vi "Main.vi"(11 "Module Admin":refnum<class "Delacor_lib_QMH_Cloneable Module Admin.lvclass">) -> ()   [LabVIEW 2020, in "Client HTTP Post.lvlib"]
doc: "This template is based off of the Queued Message Handler design pattern and the Queued Message Handler project template that ships with LabVIEW.\n\nThe main difference is that the queue is private to this module and communication between modules is performed via Broadcast and Request events.\n\nRequest events are wrapped in public API methods and are handled in the Event Handling Loop (EHL) of this VI. Any module can register for Broadcast events sent by this module. The EHL generates messages based on user interface actions.\n\nThe Message Handling Loop (MHL) processes messages generated by the EHL, or by other messages. The messages are string values, so new messages can be added easily to the Message Cases case structure in the MHL. Each message cluster can also provide an optional value for Message Data, which is a variant that can be converted to whatever message-specific data is required.\n_____\nBased on DQMH Project Template 6.0.0.91."
uses:
  Client HTTP Post.lvlib
  <vilib>/Delacor/Delacor QMH/Libraries/Cloneable Module Admin_class/Delacor_lib_QMH_Cloneable Module Admin.lvclass
  C:/Program Files (x86)/National Instruments/LabVIEW 2020/vi.lib/Delacor/Delacor QMH/Libraries/Module Admin_class/Delacor_lib_QMH_Module Admin.lvclass
  Module Data--cluster.ctl
  Do Something Argument--cluster.ctl
  <vilib>/Delacor/Delacor QMH/Libraries/Message Queue_class/Delacor_lib_QMH_Message Queue.lvclass/Delacor_lib_QMH_Message Queue.ctl
  Do Something Else Argument--cluster.ctl
  Do Something Else and Wait for Reply Argument--cluster.ctl
  Do Something Else and Wait (Reply Payload)--cluster.ctl
  <vilib>/Delacor/Delacor QMH/Libraries/Cloneable Module Admin_class/Delacor_lib_QMH_Cloneable Module Admin.lvclass/Delacor_lib_QMH_Cloneable Module Admin.ctl
  Stop Argument--cluster.ctl
  <vilib>/Delacor/Delacor QMH/Libraries/Module Admin_class/Delacor_lib_QMH_Module Admin.lvclass/Delacor_lib_QMH_Module Admin.ctl
  <vilib>/Delacor/Delacor QMH/Libraries/Message Queue_class/Delacor_lib_QMH_Enqueue Message (Single).vi
  <vilib>/Delacor/Delacor QMH/Libraries/Cloneable Module Admin_class/Delacor_lib_QMH_Get Module ID.vi
  <vilib>/Delacor/Delacor QMH/Libraries/Module Admin_class/Delacor_lib_QMH_Get External Launch.vi
  <vilib>/httpClient/POSTBuffer.vi
  <vilib>/Utility/error.llb/Error Cluster From Error Code.vi
  <vilib>/ErrorRing/Error Ring.xnode
  <vilib>/Delacor/Delacor QMH/Libraries/Message Queue_class/Delacor_lib_QMH_Message Queue.lvclass
  Hardware DAQ/Hardware DAQ.lvlib
  <vilib>/httpClient/LabVIEWHTTPClient.lvlib
panel:
  out "Array Data Termocuple & Voltage":dbl[](array[numeric])
  in  "Enviar":bool
  in  "Variables":enum16{"1 Variable", "Mas de una Variable"}(ring)
  out "body":string
  out "headers":string
  in  "POST":T1={"URL"="things.ubidots.com/api/v1.6/devices/system_daq", "Nombre - Variable"="signal", "Token"="BBFF-FQubfN2B9slUP8xWYB99mULTCcM9aX"}
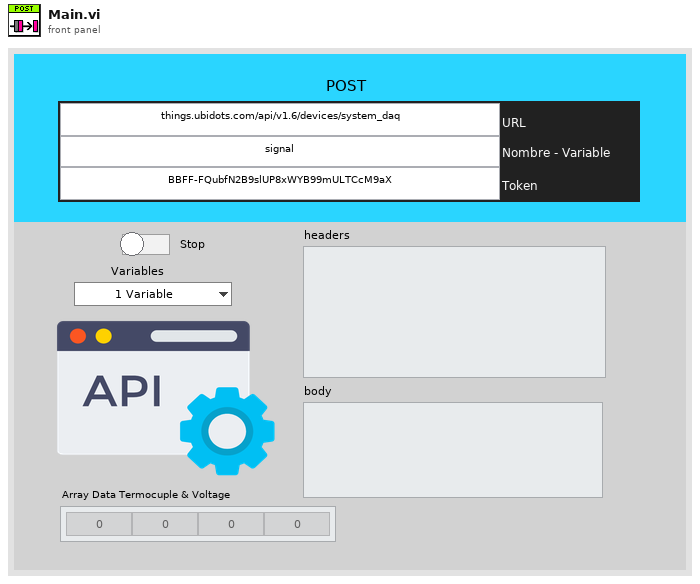
[diagram p1: front panel]
types:
  T1 = cluster{"URL":string, "Nombre - Variable":string, "Token":string}
  T2 = typedef "Client HTTP Post.lvlib/Request Events--cluster.ctl" = cluster{"Stop Module":refnum<user-event>, "Do Something":refnum<user-event>, "Do Something Else":refnum<user-event>, "Do Something Else and Wait for Reply":refnum<user-event>, "Show Panel":refnum<user-event>, "Hide Panel":refnum<user-event>, "Show Diagram":refnum<user-event>, "Get Module Execution Status":refnum<user-event>}
  T3 = typedef "Hardware DAQ.lvlib/Broadcast Events--cluster.ctl" = cluster{"Module Did Init":refnum<user-event>, "Status Updated":refnum<user-event>, "Error Reported":refnum<user-event>, "Module Did Stop":refnum<user-event>, "Update Module Execution Status":refnum<user-event>, "Hardware Connected":refnum<user-event>, "Data Process Volt":refnum<user-event>, "Coil values":refnum<user-event>}
  T4 = typedef "Client HTTP Post.lvlib/Module Data--cluster.ctl" = cluster{"Status":string}
  T5 = typedef "Client HTTP Post.lvlib/Do Something Argument--cluster.ctl" = cluster{"Module ID":i32, "Do Something Msg":string}
  T6 = typedef "Client HTTP Post.lvlib/Do Something Else Argument--cluster.ctl" = cluster{"Module ID":i32, "Do Something Else Msg":string, "X":dbl}
  T7 = typedef "Client HTTP Post.lvlib/Do Something Else and Wait for Reply Argument--cluster.ctl" = cluster{"Module ID":i32, "Do Something Else Msg":string, "X":dbl, "Wait Notifier":refnum<notifier>, "wait for reply":bool}
  T8 = enum32{"invalid lock state", "Not Locked", "Locked (No Password)", "Password-protected"}
  T9 = typedef "Client HTTP Post.lvlib/Stop Argument--cluster.ctl" = cluster{"Module ID":i32, "Origin":string, "Exit via Stop Module Req?":bool, "Wait for Module to stop?":bool}
  T10 = enum32{"Invalid", "Standard", "Closed", "Hidden", "Minimized", "Maximized"}
  T11 = cluster{"POST":cluster{"URL":string, "Nombre - Variable":string, "Token":string}, "Data Process.Volt":dbl[]}
  T12 = typedef "Client HTTP Post.lvlib/Do Something Else and Wait (Reply Payload)--cluster.ctl" = cluster{"Value":dbl, "error":errorcluster}
  T13 = typedef "LabVIEWHTTPClient.lvlib/ClientHandle.ctl" = refnum<k1>
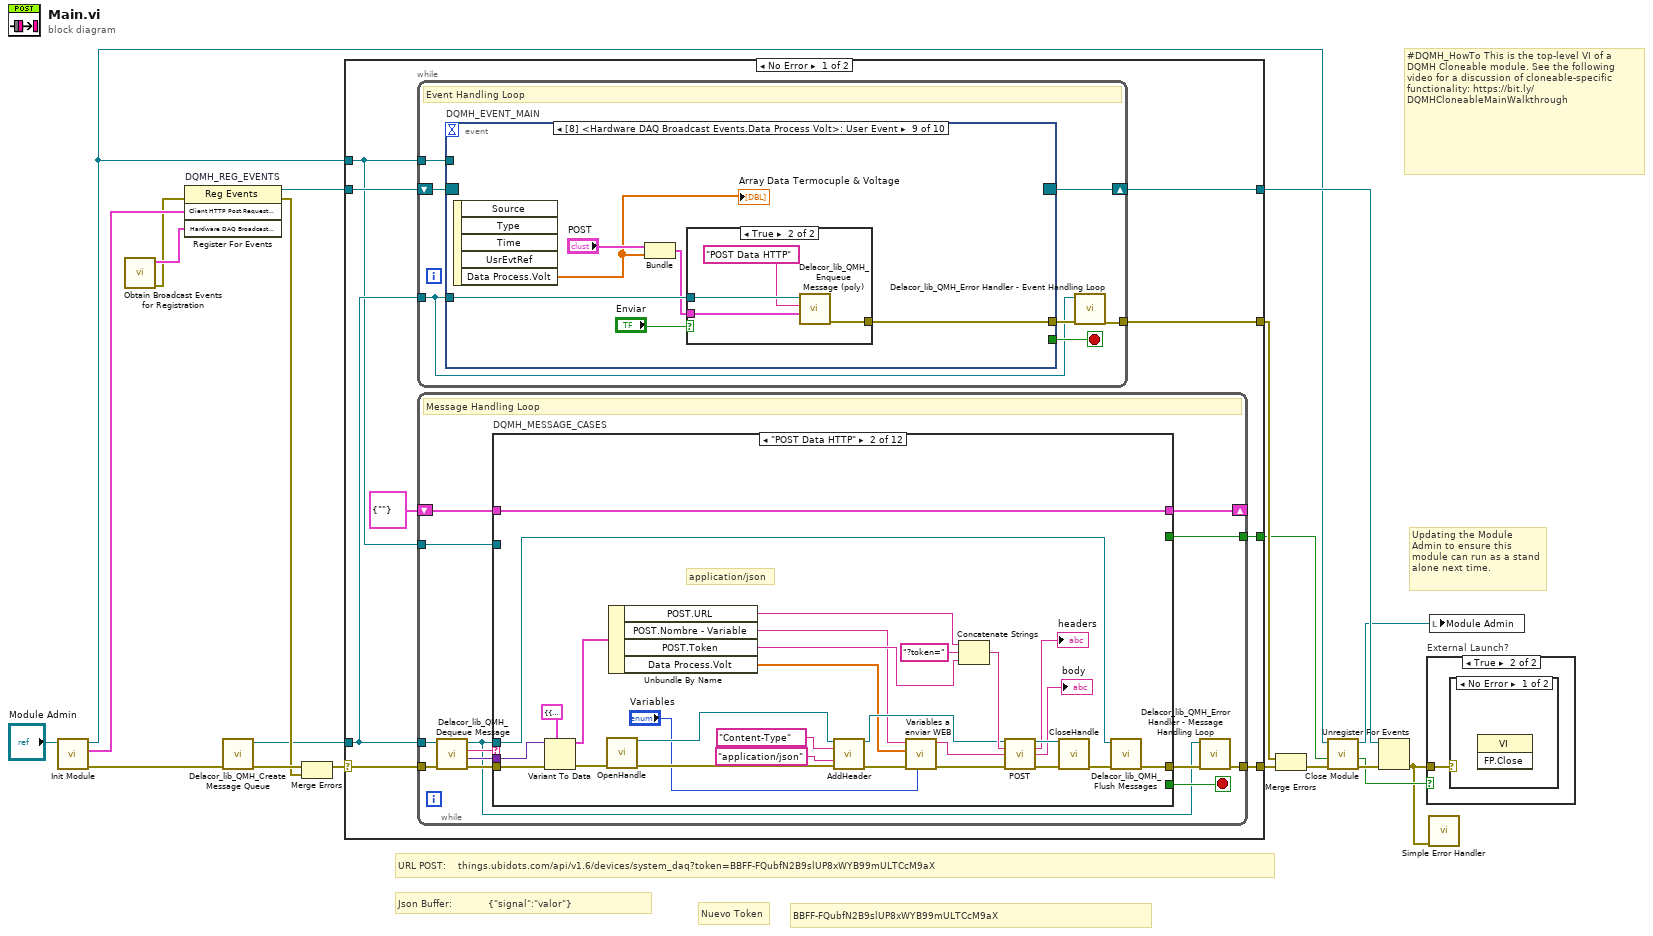
[diagram p0: block diagram]
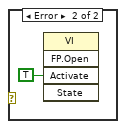
[diagram p3: hidden frame]
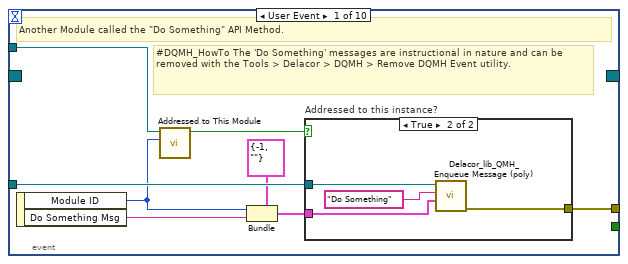
[diagram p4: hidden frame]
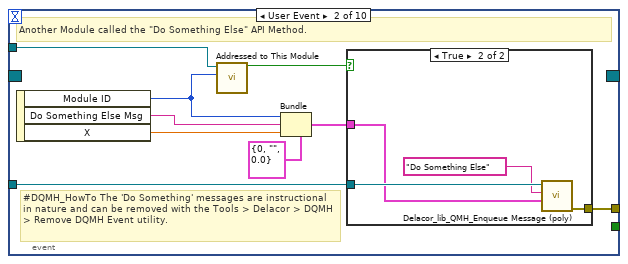
[diagram p6: hidden frame]
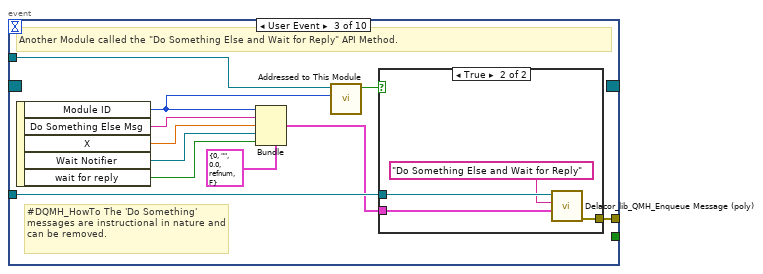
[diagram p8: hidden frame]
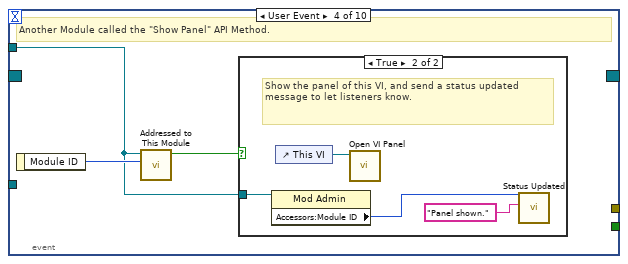
[diagram p10: hidden frame]
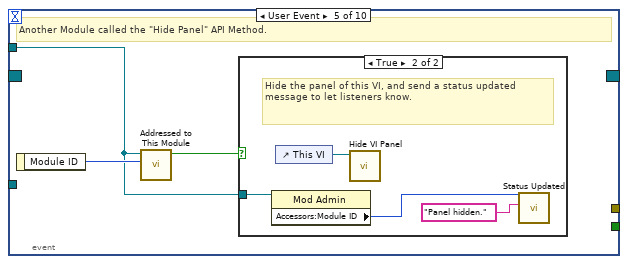
[diagram p12: hidden frame]
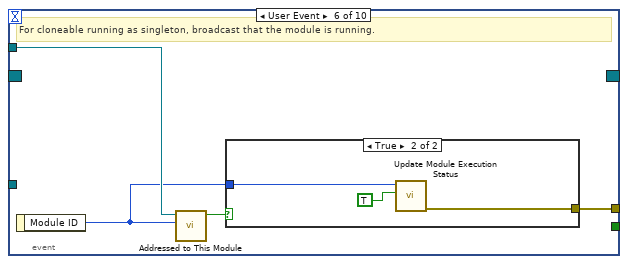
[diagram p14: hidden frame]
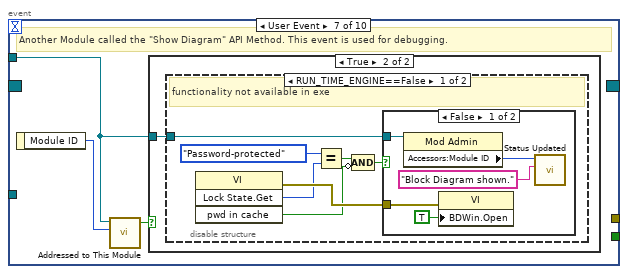
[diagram p16: hidden frame]
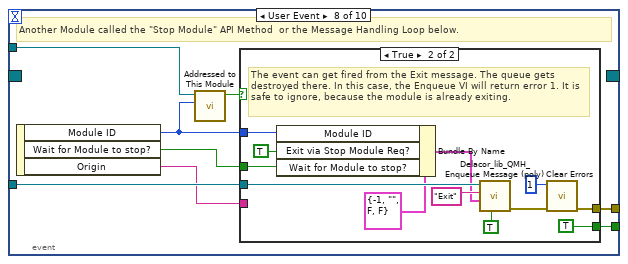
[diagram p20: hidden frame]
diagram:
  # "BBFF-FQubfN2B9slUP8xWYB99mULTCcM9aX"
  # "Nuevo Token"
  # "URL POST:    things.ubidots.com/api/v1.6/devices/system_daq?token=BBFF-FQubfN2B9slUP8xWYB99mULTCcM9aX"
  # "Json Buffer:            {\"signal\":\"valor\"}"
  # "#DQMH_HowTo This is the top-level VI of a DQMH Cloneable module. See the following video for a discussion of cloneable-specific functionality: https://bit.ly/DQMHCloneableMainWalkthrough"
  # "Updating the Module Admin to ensure this module can run as a stand alone next time."
  n1 = call "Init Module.vi"("Cloneable Module Admin in"="Module Admin") -> ("error out"=w17:errorcluster, "Client HTTP Post Request Events"=w10:T2, "Cloneable Module Admin out"=w7:refnum<class "Delacor_lib_QMH_Cloneable Module Admin.lvclass">)  [unwired: 8 in]
  n2 = call "Obtain Broadcast Events for Registration.vi"() -> ("error out"=w1:errorcluster, "Hardware DAQ Broadcast Events"=w2:T3)  [unwired: 9 in, 1 out]
  n3 = register-events "DQMH_REG_EVENTS"(error in=w1, w10, w2) -> (reference out=w11:refnum<event-registration>, error out=w13:errorcluster)  [unwired: 1 in]
  n4 = call <vilib>:"Delacor_lib_QMH_Create Message Queue.vi"("error in"=w17) -> ("error out"=w15:errorcluster, "Message Queue"=w9:refnum<class "Delacor_lib_QMH_Message Queue.lvclass">)  [unwired: 9 in]
  n5 = Merge Errors(w15, w13) -> (w14:errorcluster)
  n6 = case shown="No Error" w14 {
    selector: w14 -> [w27 w338]
    tunnel: [w29 w337] -> w18
    tunnel: [w26 w345] -> w12
    tunnel: w11 -> [w24 w345]
    tunnel: w9 -> [w23 w336]
    tunnel: [w28 _] -> w19
    tunnel: w7 -> [w22 w341]
    tunnel: [w21 _] -> w5
    frame No Error {
      n7 = while {
        tunnel: w23 -> [w30]
        shift-right: [w33] -> w26
        shift-left: w24 -> [w34]
        tunnel: [w35] -> w28
        tunnel: w22 -> [w31]
        stop <- w32 stop-if-true
        # "Event Handling Loop"
        n8 = event "DQMH_EVENT_MAIN" shown="[8] <Hardware DAQ Broadcast Events.Data Process Volt>: User Event" {
          selector: w34 -> [_ _ _ _ _ _ _ _ _ _]
          dyn-events: [_ _ _ _ _ _ _ _ _ _] -> w33
          timeout: _ -> [_ _ _ _ _ _ _ _ _ _]
          tunnel: [_ _ _ _ _ _ _ w117 _ _] -> w32
          tunnel: w30 -> [w43 w56 w71 _ _ _ _ w120 w139 w146]
          tunnel: [w44 w57 w72 _ _ w94 _ w121 w134 w149] -> w36
          tunnel: w31 -> [w41 w54 w69 w77 w84 w92 w98 w119 _ w147]
          event User Event {
            # "#DQMH_HowTo The 'Do Something' messages are instructional in nature and can be removed with the Tools > Delacor > DQMH > Remove DQMH Event utility."
            # "Another Module called the \"Do Something\" API Method."
            n9 = event-data() -> ("Module ID"=w38:i32, "Do Something Msg"=w37:string)  [unwired: 1 in]
            n10 = call "Addressed to This Module.vi"("Module ID from Argument"=w38, "Module Admin"=w41) -> ("Addressed to this instance?"=w42:bool)  [unwired: 8 in, 1 out]
            n11 = Bundle(cluster=T5 {"Module ID"=-1, "Do Something Msg"=""} ("Do Something Argument"), "Module ID"=w38, "Do Something Msg"=w37) -> (w40:T5)
            n12 = case "Addressed to this instance?" shown="True" w42 {
              tunnel: w43 -> [_ w47]
              tunnel: [_ w48] -> w44
              tunnel: w40 -> [_ w45]
              frame False {
                # "Do nothing"
              }
              frame True {
                n13 = call-poly <vilib>:"Delacor_lib_QMH_Enqueue Message (poly).vi"("Message Data"=w45, "Message"="Do Something", "Message Queue in"=w47) -> ("error out"=w48:errorcluster)  [unwired: 7 in, 1 out]
              }
            }
          }
          event User Event {
            # "#DQMH_HowTo The 'Do Something' messages are instructional in nature and can be removed with the Tools > Delacor > DQMH > Remove DQMH Event utility."
            # "Another Module called the \"Do Something Else\" API Method."
            n14 = event-data() -> ("Module ID"=w49:i32, "Do Something Else Msg"=w50:string, "X"=w52:dbl)  [unwired: 1 in]
            n15 = call "Addressed to This Module.vi"("Module ID from Argument"=w49, "Module Admin"=w54) -> ("Addressed to this instance?"=w55:bool)  [unwired: 8 in, 1 out]
            n16 = Bundle(cluster=T6 {"Module ID"=0, "Do Something Else Msg"="", "X"=0.0} ("Do Something Else Argument"), "Module ID"=w49, "Do Something Else Msg"=w50, "X"=w52) -> (w51:T6)
            n17 = case shown="True" w55 {
              tunnel: w56 -> [_ w60]
              tunnel: [_ w61] -> w57
              tunnel: w51 -> [_ w58]
              frame False {
              }
              frame True {
                n18 = call-poly <vilib>:"Delacor_lib_QMH_Enqueue Message (poly).vi"("Message Data"=w58, "Message"="Do Something Else", "Message Queue in"=w60) -> ("error out"=w61:errorcluster)  [unwired: 7 in, 1 out]
              }
            }
          }
          event User Event {
            # "#DQMH_HowTo The 'Do Something' messages are instructional in nature and can be removed."
            # "Another Module called the \"Do Something Else and Wait for Reply\" API Method."
            n19 = event-data() -> ("Module ID"=w67:i32, "Do Something Else Msg"=w65:string, "X"=w64:dbl, "Wait Notifier"=w63:refnum<notifier>, "wait for reply"=w62:bool)  [unwired: 1 in]
            n20 = Bundle(cluster=T7 {"Module ID"=0, "Do Something Else Msg"="", "X"=0.0, "Wait Notifier"=refnum, "wait for reply"=FALSE} ("Do Something Else and Wait for Reply Argument"), "Module ID"=w67, "Do Something Else Msg"=w65, "X"=w64, "Wait Notifier"=w63, "wait for reply"=w62) -> (w66:T7)
            n21 = call "Addressed to This Module.vi"("Module ID from Argument"=w67, "Module Admin"=w69) -> ("Addressed to this instance?"=w70:bool)  [unwired: 8 in, 1 out]
            n22 = case shown="True" w70 {
              tunnel: [_ w76] -> w72
              tunnel: w71 -> [_ w75]
              tunnel: w66 -> [_ w73]
              frame False {
              }
              frame True {
                n23 = call-poly <vilib>:"Delacor_lib_QMH_Enqueue Message (poly).vi"("Message Data"=w73, "Message"="Do Something Else and Wait for Reply", "Message Queue in"=w75) -> ("error out"=w76:errorcluster)  [unwired: 7 in, 1 out]
              }
            }
          }
          event User Event {
            # "Another Module called the \"Show Panel\" API Method."
            n24 = event-data() -> ("Module ID"=w78:i32)  [unwired: 1 in]
            n25 = call "Addressed to This Module.vi"("Module ID from Argument"=w78, "Module Admin"=w77) -> ("Addressed to this instance?"=w79:bool)  [unwired: 8 in, 1 out]
            n26 = case shown="True" w79 {
              tunnel: w77 -> [_ w81]
              frame False {
              }
              frame True {
                # "Show the panel of this VI, and send a status updated message to let listeners know."
                n27 = property class="Mod Admin"(reference=w81) -> ("Accessors:Module ID"=w80:i32)  [unwired: 1 in, 2 out]
                n28 = control-ref of="This VI"() -> (w83:refnum<vi>)
                n29 = call "Open VI Panel.vi"("VI"=w83) -> ()  [unwired: 10 in, 1 out]
                n30 = call "Status Updated.vi"("Status"="Panel shown." ("format string"), "Module ID"=w80) -> ()  [unwired: 9 in, 1 out]
              }
            }
          }
          event User Event {
            # "Another Module called the \"Hide Panel\" API Method."
            n31 = event-data() -> ("Module ID"=w85:i32)  [unwired: 1 in]
            n32 = call "Addressed to This Module.vi"("Module ID from Argument"=w85, "Module Admin"=w84) -> ("Addressed to this instance?"=w86:bool)  [unwired: 8 in, 1 out]
            n33 = case shown="True" w86 {
              tunnel: w84 -> [_ w88]
              frame False {
              }
              frame True {
                # "Hide the panel of this VI, and send a status updated message to let listeners know."
                n34 = property class="Mod Admin"(reference=w88) -> ("Accessors:Module ID"=w87:i32)  [unwired: 1 in, 2 out]
                n35 = control-ref of="This VI"() -> (w90:refnum<vi>)
                n36 = call "Hide VI Panel.vi"("VI"=w90) -> ()  [unwired: 10 in, 1 out]
                n37 = call "Status Updated.vi"("Status"="Panel hidden." ("format string"), "Module ID"=w87) -> ()  [unwired: 9 in, 1 out]
              }
            }
          }
          event User Event {
            # "For cloneable running as singleton, broadcast that the module is running."
            n38 = event-data() -> ("Module ID"=w91:i32)  [unwired: 1 in]
            n39 = call "Addressed to This Module.vi"("Module ID from Argument"=w91, "Module Admin"=w92) -> ("Addressed to this instance?"=w93:bool)  [unwired: 8 in, 1 out]
            n40 = case shown="True" w93 {
              tunnel: [_ w97] -> w94
              tunnel: w91 -> [_ w96]
              frame False {
              }
              frame True {
                n41 = call "Update Module Execution Status.vi"("Running?"=TRUE, "Module ID"=w96) -> ("error out"=w97:errorcluster)  [unwired: 9 in]
              }
            }
          }
          event User Event {
            # "Another Module called the \"Show Diagram\" API Method. This event is used for debugging."
            n42 = event-data() -> ("Module ID"=w99:i32)  [unwired: 1 in]
            n43 = call "Addressed to This Module.vi"("Module ID from Argument"=w99, "Module Admin"=w98) -> ("Addressed to this instance?"=w100:bool)  [unwired: 8 in, 1 out]
            n44 = case shown="True" w100 {
              tunnel: w98 -> [_ w101]
              frame False {
              }
              frame True {
                n45 = disable-structure shown="RUN_TIME_ENGINE==False" {
                  disable-tunnel: w101 -> [w102 _]
                  frame condition #0 (active) {
                    # "functionality not available in exe"
                    n46 = invoke class="VI" method="Lock State.Get"() -> (error out=w108:errorcluster, "Get Lock State"=w107:T8, "pwd in cache"=w104:bool)  [unwired: 4 in, 1 out]
                    n47 = Equal?(x=T8."Password-protected", y=w107) -> (x = y?=w105:bool)
                    n48 = Compound Arithmetic op=AND(w105, invert w104) -> (w103:bool)
                    n49 = case shown="False" w103 {
                      tunnel: w108 -> [w113 _]
                      tunnel: w102 -> [w110 _]
                      frame False {
                        n50 = property class="Mod Admin"(reference=w110) -> ("Accessors:Module ID"=w109:i32)  [unwired: 1 in, 2 out]
                        n51 = property class="VI"(error in=w113, "BDWin.Open"=TRUE ("Block Diagram Window:Open")) -> ()  [unwired: 1 in, 2 out]
                        n52 = call "Status Updated.vi"("Status"="Block Diagram shown." ("format string"), "Module ID"=w109) -> ()  [unwired: 9 in, 1 out]
                      }
                      frame True {
                        # "Password-protected VI, and the password is not in the cache. Do not show the diagram."
                      }
                    }
                  }
                  frame condition #1 {
                  }
                }
              }
            }
          }
          event User Event {
            # "Another Module called the \"Stop Module\" API Method  or the Message Handling Loop below."
            n53 = event-data() -> ("Module ID"=w115:i32, "Wait for Module to stop?"=w116:bool, "Origin"=w114:string)  [unwired: 1 in]
            n54 = call "Addressed to This Module.vi"("Module ID from Argument"=w115, "Module Admin"=w119) -> ("Addressed to this instance?"=w118:bool)  [unwired: 8 in, 1 out]
            n55 = case shown="True" w118 {
              tunnel: [_ w132] -> w121
              tunnel: w120 -> [_ w128]
              tunnel: [_ TRUE] -> w117
              tunnel: w116 -> [_ w123]
              tunnel: w115 -> [_ w125]
              tunnel: w114 -> [_ _]
              frame False {
              }
              frame True {
                # "The event can get fired from the Exit message. The queue gets destroyed there. In this case, the Enqueue VI will return error 1. It is safe to ignore, because the module is already exiting."
                n56 = Bundle By Name(cluster=T9 {"Module ID"=-1, "Origin"="", "Exit via Stop Module Req?"=FALSE, "Wait for Module to stop?"=FALSE} ("Stop Argument"), "Module ID"=w125, "Exit via Stop Module Req?"=TRUE, "Wait for Module to stop?"=w123) -> (w122:T9)
                n57 = call-poly <vilib>:"Delacor_lib_QMH_Enqueue Message (poly).vi"("Priority Message? (F)"=TRUE, "Message Data"=w122, "Message"="Exit", "Message Queue in"=w128) -> ("error out"=w133:errorcluster)  [unwired: 6 in, 1 out]
                n58 = call <vilib>:"Clear Errors.vi"("error in (no error)"=w133, "specific error code to clear (0: all)"=1) -> ("error out"=w132:errorcluster)  [unwired: 4 in, 1 out]
              }
            }
          }
          event User Event {
            n59 = event-data() -> ("Data Process.Volt"=w135:dbl[])  [unwired: 1 in, 4 out]
            "Array Data Termocuple & Voltage" <- w135
            n60 = Bundle("POST"="POST", "Data Process.Volt"=w135) -> (w136:T11)  [unwired: 1 in]
            n61 = case shown="True" "Enviar" {
              tunnel: w139 -> [_ w144]
              tunnel: [errorcluster {"status"=FALSE, "code"=0, "source"=""} ("error out") w143] -> w134
              tunnel: w136 -> [_ w141]
              frame False {
              }
              frame True {
                n62 = call-poly <vilib>:"Delacor_lib_QMH_Enqueue Message (poly).vi"("Message Data"=w141, "Message"="POST Data HTTP", "Message Queue in"=w144) -> ("error out"=w143:errorcluster)  [unwired: 7 in, 1 out]
              }
            }
          }
          event Panel Close? {
            w148 = TRUE  # Discard the event, the MHL is responsible for closing and stopping this VI.
            # "Hide the panel or send the 'Exit' message if the user clicks the 'X' on the module main VI panel."
            n63 = event-data() -> ()  [unwired: 1 in, 1 out]
            n64 = property class="Mod Admin"(reference=w147) -> ("Accessors:External Launch"=w145:bool)  [unwired: 1 in, 2 out]
            n65 = case shown="True" w145 {
              tunnel: w146 -> [_ w153]
              tunnel: [_ w154] -> w149
              frame True {
                # "If externally launched, clicking the 'X' hides the panel, but doesn't close it."
                n66 = control-ref of="This VI"() -> (w150:refnum<vi>)
                n67 = call "Hide VI Panel.vi"("VI"=w150) -> ()  [unwired: 10 in, 1 out]
              }
              frame False {
                # "If run as a stand-alone VI, clicking the panel 'X' stops the VI."
                n68 = call-poly <vilib>:"Delacor_lib_QMH_Enqueue Message (poly).vi"("Priority Message? (F)"=TRUE, "Message"="Exit", "Message Queue in"=w153) -> ("error out"=w154:errorcluster)  [unwired: 7 in, 1 out]
              }
            }
            n69 = event-data("Discard?"=w148) -> ()  [unwired: 1 in, 1 out]
          }
        }
        n70 = call-dynamic "Delacor_lib_QMH_Error Handler - Event Handling Loop.vi"("error in"=w36, "Message Queue in"=w30) -> ("dup error in"=w35:errorcluster)  [unwired: 8 in, 1 out]
      }
      n71 = while {
        tunnel: w23 -> [w158]
        shift-right: [w162] -> _
        shift-left: T4 {"Status"=""} ("Data Cluster") -> [w163]
        tunnel: w27 -> [w166]
        tunnel: [w164] -> w29
        tunnel: w22 -> [w156]
        tunnel: [w155] -> w21
        stop <- w161 stop-if-true
        # "Message Handling Loop"
        n72 = call-dynamic "Delacor_lib_QMH_Dequeue Message.vi"("error in"=w166, "Message Queue in"=w158) -> ("error out"=w165:errorcluster, "Message Data"=w159:variant, "Message"=w160:string, "Message Queue out"=w157:refnum<class "Delacor_lib_QMH_Message Queue.lvclass">)  [unwired: 6 in]
        n73 = case "DQMH_MESSAGE_CASES" shown="\"POST Data HTTP\"" w160 {
          selector: w160 -> [_ _ _ _ _ _ _ _ _ _ _ w323]
          tunnel: w157 -> [_ w186 _ _ _ _ _ _ w275 _ w313 _]
          tunnel: w165 -> [w182 w198 w213 w223 w234 w255 w270 w272 w283 w296 w319 w325]
          tunnel: [w180 w184 w213 w221 w224 w254 w269 w272 w273 w295 w316 w326] -> w167
          tunnel: w163 -> [w168 w211 w212 w220 w233 w252 w268 w271 w279 w293 w312 w324]
          tunnel: [w168 w211 w212 w220 w233 w252 w268 w271 w279 w293 w312 w324] -> w162
          tunnel: [_ _ _ _ _ _ _ _ _ _ w311 _] -> w161
          tunnel: w159 -> [_ w191 _ w219 w230 w249 _ _ w278 _ w309 _]
          tunnel: w156 -> [w170 _ _ w215 w226 w239 _ _ w277 w291 w305 w321]
          tunnel: [_ _ _ _ _ _ _ _ _ _ w307 _] -> w155
          frame "Initialize" {
            # "Initialize - Any operation that needs to be done before the module can receive messages. Synchronize Caller Events.vi will inform Start Module.vi that the module has launched and is ready to receive messages. Module Did Init.vi will broadcast that the module initialized."
            n74 = call "Synchronize Caller Events.vi"("error in (no error)"=w182, "Module Admin"=w170) -> ("error out"=w181:errorcluster, "Module Admin out"=w169:refnum<class "Delacor_lib_QMH_Cloneable Module Admin.lvclass">)  [unwired: 8 in]
            n75 = property class="Mod Admin"(reference=w169) -> ("Accessors:Module ID"=w172:i32, "Accessors:External Launch"=w171:bool)  [unwired: 1 in, 2 out]
            n76 = call "Module Name--constant.vi"("Module ID"=w172) -> ("Module Name"=w178:string)  [unwired: 10 in]
            n77 = property class="VI"("Front Panel.Title"=w178) -> (reference out=w179:refnum<vi>, error out=w183:errorcluster)  [unwired: 2 in]
            n78 = Select(t=T10."Hidden" ("State"), s=w171, f=T10."Standard" ("State")) -> (s? t:f=w175:T10)
            n79 = invoke class="VI" method="FP.Open"(reference=w179, error in=w183, "State"=w175) -> ()  [unwired: 2 in, 5 out]
            n80 = call "Module Name--constant.vi"("Module ID"=w172) -> ("Module Name"=w173:string)  [unwired: 10 in]
            n81 = call "Module Did Init.vi"("error in (no error)"=w181, "Initialized?"=TRUE, "Origin"=w173, "Module ID"=w172) -> ("error out"=w180:errorcluster)  [unwired: 7 in]
          }
          frame "POST Data HTTP" {
            # "application/json"
            n82 = Variant To Data(error in=w198, type=T11 {"POST"={"URL"="", "Nombre - Variable"="", "Token"=""}, "Data Process.Volt"=[]} ("output cluster"), Variant=w191) -> (data=w203:T11, error out=w208:errorcluster)
            n83 = call <vilib>:"OpenHandle.vi"("error in (no error)"=w208) -> ("client handle out"=w210:T13, "error out"=w209:errorcluster)  [unwired: 13 in]
            n84 = Unbundle By Name(w203) -> ("POST.URL"=w205:string, "POST.Nombre - Variable"=w194:string, "POST.Token"=w206:string, "Data Process.Volt"=w189:dbl[])
            n85 = call <vilib>:"AddHeader.vi"("client handle"=w210, "header"="Content-Type", "value"="application/json", "error in (no error)"=w209) -> ("client handle out"=w204:T13, "error out"=w197:errorcluster)  [unwired: 10 in]
            n86 = call "Variables a enviar WEB.vi"("#Variables"="Variables", "error in"=w197, "Array Data"=w189, "Nombre Variable"=w194) -> ("error out"=w196:errorcluster, "Trama Json"=w195:string)  [unwired: 6 in]
            n87 = Concatenate Strings(w205, "?token=" ("string"), w206) -> (w207:string)
            n88 = call-poly <vilib>:"POST.vi"("client handle"=w204, "url"=w207, "buffer"=w195, "error in (no error)"=w196) -> ("client handle out"=w192:T13, "headers"=→"headers":string, "body"=→"body":string, "error out"=w193:errorcluster)  [unwired: 8 in]
            n89 = call <vilib>:"CloseHandle.vi"("client handle"=w192, "error in (no error)"=w193) -> ("error out"=w185:errorcluster)  [unwired: 13 in]
            n90 = call-dynamic "Delacor_lib_QMH_Flush Messages.vi"("error in"=w185, "Message Queue in"=w186) -> ("error out"=w184:errorcluster)  [unwired: 6 in, 3 out]
          }
          frame "---Module Specific---" {
            # "Separator -- The following cases handle messages specific to this Module."
          }
          frame "Do Something" {
            # "#DQMH_HowTo The 'Do Something' messages are instructional in nature and can be removed with the Tools > Delacor > DQMH > Remove DQMH Event utility."
            # "Do Something - Replace this message with functionality for your own application. Note that this message also fires the \"Did Something\" broadcast event."
            n91 = Variant To Data(error in=w223, type=T5 {"Module ID"=-1, "Do Something Msg"=""} ("Do Something Argument"), Variant=w219) -> (data=w218:T5, error out=w222:errorcluster)
            n92 = property class="Mod Admin"(reference=w215) -> ("Accessors:Module ID"=w214:i32)  [unwired: 1 in, 2 out]
            n93 = Unbundle By Name(w218) -> ("Do Something Msg"=w216:string)
            n94 = call "Status Updated.vi"("Status"=w216, "Module ID"=w214) -> ()  [unwired: 9 in, 1 out]
            n95 = call "Did Something.vi"("error in (no error)"=w222, "Did Something Msg"=w216, "Module ID"=w214) -> ("error out"=w221:errorcluster)  [unwired: 8 in]
          }
          frame "Do Something Else" {
            # "#DQMH_HowTo The 'Do Something' messages are instructional in nature and can be removed with the Tools > Delacor > DQMH > Remove DQMH Event utility."
            # "Do Something Else - Replace this message with functionality for your own application."
            n96 = Variant To Data(error in=w234, type=T6 {"Module ID"=0, "Do Something Else Msg"="", "X"=0.0} ("Do Something Else Argument"), Variant=w230) -> (data=w231:T6, error out=w224:errorcluster)
            n97 = Unbundle By Name(w231) -> ("Do Something Else Msg"=w229:string, "X"=w228:dbl)
            n98 = property class="Mod Admin"(reference=w226) -> ("Accessors:Module ID"=w225:i32)  [unwired: 1 in, 2 out]
            n99 = Format Into String(initial string=w229, w228) -> (resulting string=w227:string)  [unwired: 2 in, 1 out]
            n100 = call "Status Updated.vi"("Status"=w227, "Module ID"=w225) -> ()  [unwired: 9 in, 1 out]
          }
          frame "Do Something Else and Wait for Reply" {
            w242 = "X(%.2f)+Offset(%.2f)=%.2f"  # status message format string
            # "#DQMH_HowTo The 'Do Something' messages are instructional in nature and can be removed."
            # "Send back X with a random offset"
            # "Do Something Else and Wait for Reply - Replace this message with functionality for your own application. Note that this message must fire a notifier to let callers know it has finished execution, and it returns an error if the 'Value' is negative."
            n101 = Variant To Data(error in=w255, type=T7 {"Module ID"=0, "Do Something Else Msg"="", "X"=0.0, "Wait Notifier"=refnum, "wait for reply"=FALSE} ("Do Something Else and Wait for Reply Argument"), Variant=w249) -> (data=w250:T7, error out=w236:errorcluster)
            n102 = Unbundle By Name(w250) -> ("Wait Notifier"=w247:refnum<notifier>, "Do Something Else Msg"=w248:string, "X"=w244:dbl, "wait for reply"=w235:bool)
            n103 = property class="Mod Admin"(reference=w239) -> ("Accessors:Module ID"=w238:i32)  [unwired: 1 in, 2 out]
            n104 = Random Number (0-1)() -> (number: 0 to 1=w243:dbl)
            n105 = Add(x=w243, y=w244) -> (x+y=w237:dbl)
            n106 = Format Into String(format string=w242, initial string=w248, w244, w243, w237) -> (resulting string=w240:string)  [unwired: 1 in, 1 out]
            n107 = Less Than 0?(x=w237) -> (x < 0?=w241:bool)
            n108 = case shown="True" w241 {
              tunnel: [_ w262] -> w253
              frame False {
              }
              frame True {
                n109 = xnode "Error Ring"() -> ("error out"=w262:errorcluster)
              }
            }
            n110 = Bundle By Name(cluster=T12 {"Value"=0.0, "error"={"status"=FALSE, "code"=0, "source"=""}} ("notification"), "error"=w253, "Value"=w237) -> (w245:T12)
            n111 = call "Status Updated.vi"("Status"=w240, "Module ID"=w238) -> ()  [unwired: 9 in, 1 out]
            n112 = case shown="True" w235 {
              tunnel: w247 -> [_ w259]
              tunnel: w245 -> [_ w258]
              frame False {
              }
              frame True {
                # "Simulate an operation that requires a wait."
                n113 = Wait (ms)(milliseconds to wait=u32 1000) -> (millisecond timer value=w256:u32)
                n114 = flat-sequence {
                  tunnel: w259 -> [w261]
                  tunnel: w258 -> [w260]
                  tunnel: w256 -> [_]
                  frame #0 {
                    n115 = Send Notification(notification=w260, notifier=w261) -> ()  [unwired: 1 in, 2 out]
                  }
                }
              }
            }
            n116 = Merge Errors(w236, w253) -> (w254:errorcluster)
          }
          frame "---Copy This Frame---" {
            # "Duplicate this frame when creating new messages.  Change this comment in the duplicated frame to describe this message."
            n117 = Merge Errors(w270) -> (w269:errorcluster)
          }
          frame "---Exit and Error Handling---" {
            # "Separator - the following cases handle errors and exit messages."
          }
          frame "Error" {
            # "Error - Check the error message data and respond accordingly. This message is sent by the \"Error Handler\" VIs at the end of each loop in this application."
            n118 = property class="Mod Admin"(reference=w277) -> ("Accessors:External Launch"=w276:bool, "Accessors:Module ID"=w274:i32)  [unwired: 1 in, 2 out]
            n119 = Variant To Data(error in=w283, type=errorcluster {"status"=FALSE, "code"=0, "source"=""} ("error constant"), Variant=w278) -> (data=w284:errorcluster, error out=w281:errorcluster)
            n120 = call "Error Reported.vi"("Error"=w284, "Module ID"=w274) -> ()  [unwired: 9 in, 1 out]
            n121 = case shown="False" w276 {
              tunnel: [w289 _] -> w280
              tunnel: w275 -> [w287 _]
              tunnel: w284 -> [w288 _]
              frame False {
                # "If the module is running standalone, then pop up an error dialog and call the \"Exit\" message."
                n122 = call <vilib>:"Simple Error Handler.vi"("error in (no error)"=w288) -> ()  [unwired: 4 in, 5 out]
                n123 = call-poly <vilib>:"Delacor_lib_QMH_Enqueue Message (poly).vi"("Priority Message? (F)"=TRUE, "Message"="Exit", "Message Queue in"=w287) -> ("error out"=w289:errorcluster)  [unwired: 7 in, 1 out]
              }
              frame True {
                # "If the module was launched externally, calling the Error Reported broadcast VI is the only action performed by the \"Error\" message. The module's caller can then process the error appropriately."
              }
            }
            n124 = Merge Errors(w281, w280) -> (w273:errorcluster)
            n125 = call <vilib>:"Simple Error Handler.vi"("error in (no error)"=w273) -> ()  [unwired: 4 in, 5 out]
          }
          frame "Simulate MHL Error" {
            # "#DQMH_HowTo The 'Simulate MHL Error' button  illustrates how the MHL handles errors. This event is instructional in nature and can be removed."
            # "Simulate an error occurring at the MHL"
            n126 = property class="Mod Admin"(reference=w291) -> ("Accessors:Module ID"=w292:i32)  [unwired: 1 in, 2 out]
            n127 = call "Module Name--constant.vi"("Module ID"=w292) -> ("Module Name"=w290:string)  [unwired: 10 in]
            n128 = xnode "Error Ring"("parameter 0"=w290) -> ("error out"=w294:errorcluster)
            n129 = Merge Errors(w296, w294) -> (w295:errorcluster)
          }
          frame "Exit" {
            w310 = 91  # 91: not all Exit messages will have an argument
            w311 = TRUE  # Stop the VI
            # "Release the message queue reference"
            # "#CodeNeeded - Add any required cleanup code here."
            # "Exit - Exit the application."
            n130 = Variant To Data(error in=w319, type=T9 {"Module ID"=-1, "Origin"="", "Exit via Stop Module Req?"=FALSE, "Wait for Module to stop?"=FALSE} ("Stop Argument"), Variant=w309) -> (data=w306:T9, error out=w314:errorcluster)
            n131 = call <vilib>:"Clear Errors.vi"("error in (no error)"=w314, "specific error code to clear (0: all)"=w310) -> ("error out"=w318:errorcluster)  [unwired: 4 in, 1 out]
            n132 = control-ref of="This VI"() -> (w304:refnum<vi>)
            n133 = call-dynamic "Delacor_lib_QMH_Release Message Queue.vi"("error in"=w318, "Message Queue"=w313) -> ("error out"=w317:errorcluster)  [unwired: 9 in]
            n134 = call "Handle Exit.vi"("Stop Argument"=w306, "Module Admin in"=w305, "VI reference"=w304) -> ("error out"=w315:errorcluster, "Wait for Stop?"=w307:bool)  [unwired: 7 in]
            n135 = Merge Errors(w317, w315) -> (w316:errorcluster)
          }
          frame Default {
            # "'Default' case only runs if there is a message that isn't defined in any of the other cases.  Output a programming error."
            n136 = property class="Mod Admin"(reference=w321) -> ("Accessors:Module ID"=w320:i32)  [unwired: 1 in, 2 out]
            n137 = call "Module Name--constant.vi"("Module ID"=w320) -> ("Module Name"=w322:string)  [unwired: 10 in]
            n138 = xnode "Error Ring"("parameter 0"=w323, "parameter 1"=w322) -> ("error out"=w327:errorcluster)
            n139 = Merge Errors(w325, w327) -> (w326:errorcluster)
          }
        }
        n140 = call-dynamic "Delacor_lib_QMH_Error Handler - Message Handling Loop.vi"("error in"=w167, "Message Queue in"=w157) -> ("dup error in"=w164:errorcluster)  [unwired: 8 in, 1 out]
      }
    }
    frame Error {
      n141 = call "Synchronize Caller Events.vi"("Module Admin"=w341) -> ("Module Admin out"=w340:refnum<class "Delacor_lib_QMH_Cloneable Module Admin.lvclass">)  [unwired: 9 in, 1 out]
      n142 = property class="Mod Admin"(reference=w340) -> ("Accessors:Module ID"=w339:i32)  [unwired: 1 in, 2 out]
      n143 = call-dynamic "Delacor_lib_QMH_Release Message Queue.vi"("error in"=w338, "Message Queue"=w336) -> ("error out"=w337:errorcluster)  [unwired: 9 in]
      n144 = call "Module Name--constant.vi"("Module ID"=w339) -> ("Module Name"=w344:string)  [unwired: 10 in]
      n145 = Format Into String(format string="An error occurred during initialization. %s is no longer running.", w344) -> (resulting string=w342:string)  [unwired: 2 in, 1 out]
      n146 = call "Error Reported.vi"("Additional Information"=w342, "Error"=w337, "Module ID"=w339) -> ()  [unwired: 8 in, 1 out]
    }
  }
  n147 = Merge Errors(w19, w18) -> (w20:errorcluster)
  n148 = call "Close Module.vi"("error in"=w20, "Wait for stop?"=w5, "Module Admin in"=w7) -> ("error out"=w16:errorcluster, "External Launch"=w4:bool, "Module Admin out"=w6:refnum<class "Delacor_lib_QMH_Cloneable Module Admin.lvclass">)  [unwired: 6 in]
  n149 = Unregister For Events(event registration refnum=w12, error in=w16) -> (error out=w3:errorcluster)
  n150 = case "External Launch?" shown="True" w4 {
    tunnel: w3 -> [_ w346]
    frame False {
    }
    frame True {
      n151 = case shown="No Error" w346 {
        frame No Error {
          n152 = invoke class="VI" method="FP.Close"() -> ()  [unwired: 3 in, 3 out]
        }
        frame Error {
          n153 = invoke class="VI" method="FP.Open"("Activate"=TRUE ("Activate?")) -> ()  [unwired: 4 in, 5 out]
        }
      }
    }
  }
  n154 = call <vilib>:"Simple Error Handler.vi"("error in (no error)"=w3) -> ()  [unwired: 4 in, 5 out]
  n155 = local write "Module Admin"(w6) -> ()
